vi "Case structure in Labview.vi"() -> ()   [LabVIEW 2026]
panel:
  out "FALSE CASE - OUTPUT":dbl
  out "TRUE CASE - OUTPUT":dbl
  in  "CASE":bool
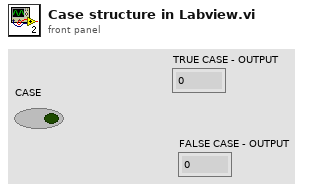
[diagram p1: front panel]
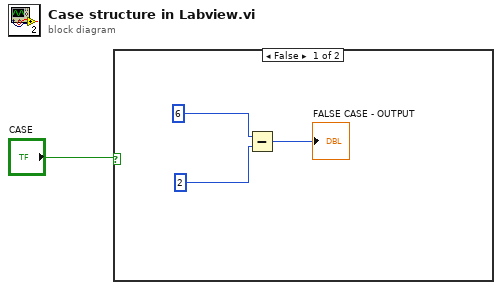
[diagram p0: block diagram]
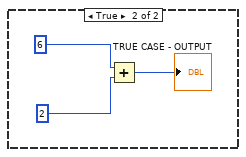
[diagram p2: hidden frame]
diagram:
  n1 = case shown="False" "CASE" {
    frame False {
      n2 = Subtract(x=6, y=2) -> (x-y=→"FALSE CASE - OUTPUT":i32)
    }
    frame True {
      n3 = Add(x=6, y=2) -> (x+y=→"TRUE CASE - OUTPUT":i32)
    }
  }
